vi "Write Lives.vi"(8 "error in (no error)":errorcluster, 10 "Lives":i16, 11 "BounceTarget in":refnum<class "BounceTarget.lvclass">) -> (0 "error out":errorcluster, 3 "BounceTarget out":refnum<class "BounceTarget.lvclass">)   [LabVIEW 2019, in "RT_Game.lvlib" / "BounceTarget.lvclass"]
uses:
  BounceTarget.lvclass
  BounceTarget.lvclass/BounceTarget.ctl
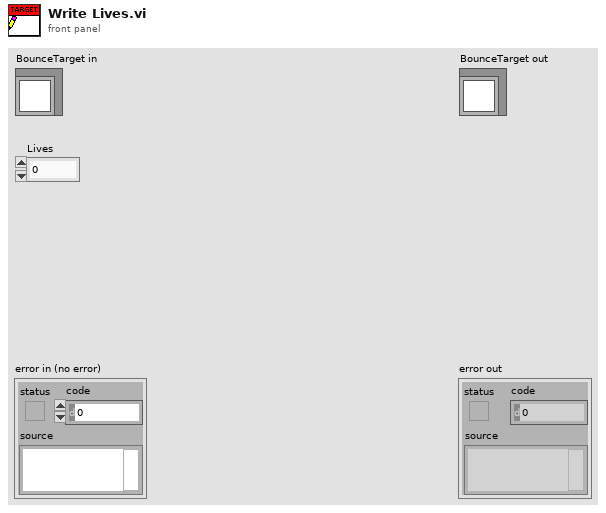
[diagram p1: front panel]
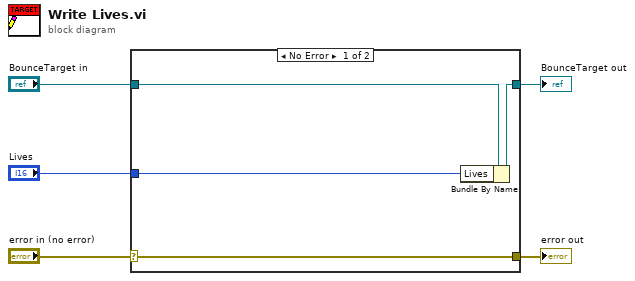
[diagram p0: block diagram]
diagram:
  n1 = case shown="No Error" "error in (no error)" {
    selector: "error in (no error)" -> [w9 w10]
    tunnel: [w9 w10] -> w4
    tunnel: [w7 w11] -> w2
    tunnel: "BounceTarget in" -> [w8 w11]
    tunnel: "Lives" -> [w6 _]
    frame No Error {
      n2 = Bundle By Name(cluster=w8, "Lives"=w6) -> (w7:refnum<class "BounceTarget.lvclass">)
    }
    frame Error {
    }
  }
  "error out" <- w4
  "BounceTarget out" <- w2
